vi "簇元素顺序.vi"() -> ()   [LabVIEW 2014]
panel:
  in  "簇":cluster{"布尔":bool, "字符串":string, "数值":dbl}
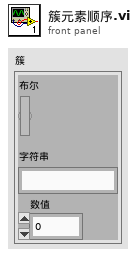
[diagram p1: front panel]
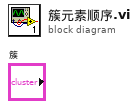
[diagram p0: block diagram]
diagram:
